vi "Actor Core.vi"(8 "error in":errorcluster, 11 "Alice in":refnum<class "Alice.lvclass">) -> (0 "error out":errorcluster, 3 "Actor out":refnum<class "Actor.lvclass">)   [LabVIEW 2014, in "Alice.lvlib" / "Alice.lvclass"]
doc: "(<B>Filename</B>: Actor Framework.lvlib:Actor.lvclass:Actor Core.vi)\n\nReceives messages to the actor, reacts to them, and initiates any error handling that may shut the actor down.\n\nDescendant classes may override this VI to append parallel tasks for the actor to complete while it handles messages. Overrides use the Call Parent Method node."
uses:
  Alice.lvclass
  <vilib>/ActorFramework/Actor/Actor.lvclass
  <vilib>/ActorFramework/Message Enqueuer/Message Enqueuer.lvclass
  Alice.lvclass/Alice.ctl
  <vilib>/ActorFramework/Actor/Actor.lvclass/Actor.ctl
  <vilib>/ActorFramework/Message Enqueuer/Message Enqueuer.lvclass/Message Enqueuer.ctl
  Proxy/Proxy Messages/Connect Msg/Connect Msg.lvclass/Connect Msg.ctl
  <vilib>/ActorFramework/Message Enqueuer/Init from Existing Queue.vi
  <vilib>/ActorFramework/Message Enqueuer/Enqueue.vi
  <vilib>/ActorFramework/Message Priority Queue/Priority Enqueue.vi
  <vilib>/ActorFramework/Stop Msg/Stop Msg.lvclass
  Bob/Bob Messages/Bob Action Msg/Bob Action Msg.lvclass
  Proxy/Proxy Messages/Connect Msg/Connect Msg.lvclass
  Proxy/Proxy Messages/Disconnect Msg/Disconnect Msg.lvclass
panel:
  in  "Disconnect":bool
  in  "Connect":bool
  in  "BobEnq":refnum<class "Message Enqueuer.lvclass">
  in  "stop 2":bool
  in  "stop":bool
  in  "Send to Bob":bool
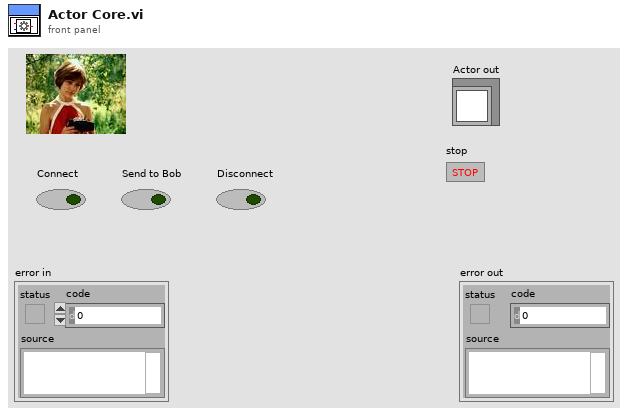
[diagram p1: front panel]
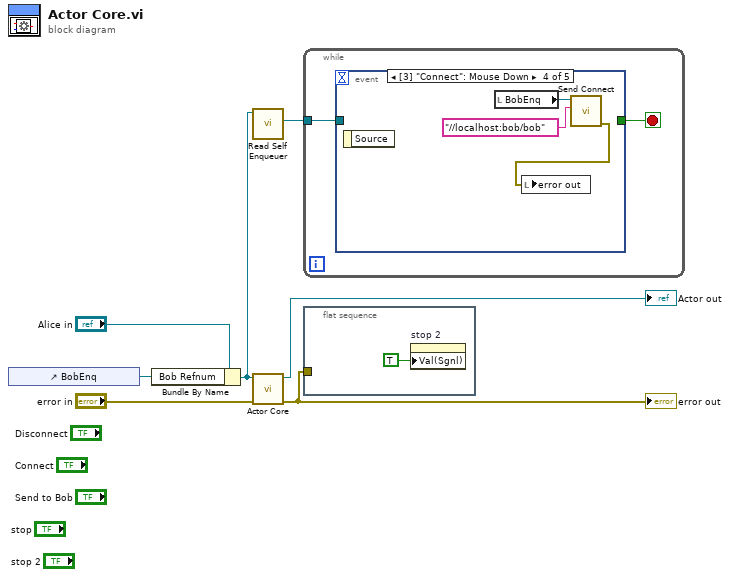
[diagram p0: block diagram]
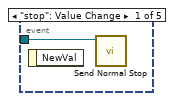
[diagram p2: hidden frame]
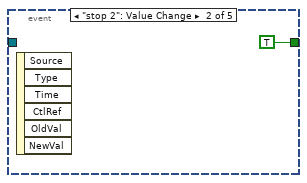
[diagram p3: hidden frame]
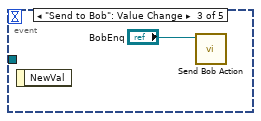
[diagram p4: hidden frame]
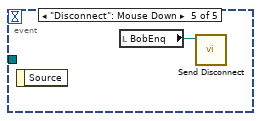
[diagram p5: hidden frame]
diagram:
  n1 = control-ref of="BobEnq"() -> (w1:refnum<vi>)
  n2 = Bundle By Name(cluster="Alice in", "Bob Refnum"=w1) -> (w2:refnum<class "Alice.lvclass">)
  n3 = call <vilib>:"Read Self Enqueuer.vi"("Actor"=w2) -> ("Self Enqueuer"=w5:refnum<class "Message Enqueuer.lvclass">)  [unwired: 10 in]
  n4 = call-parent "Actor Core.vi"("error in"="error in", "Actor in"=w2) -> ("error out"=w4:errorcluster, "Actor out"=→"Actor out":refnum<class "Actor.lvclass">)  [unwired: 8 in]
  "error out" <- w4
  n5 = while {
    tunnel: w5 -> [w9]
    stop <- w8 stop-if-true
    n6 = event shown="[3] \"Connect\": Mouse Down" {
      selector: _ -> [_ _ _ _ _]
      dyn-events: _ -> [_ _ _ _ _]
      timeout: _ -> [_ _ _ _ _]
      tunnel: w9 -> [w10 _ _ _ _]
      tunnel: [_ TRUE _ _ _] -> w8
      event "stop": Value Change {
        n7 = event-data() -> ()  [unwired: 1 in, 1 out]
        n8 = call <vilib>:"Send Normal Stop.vi"("Message Enqueuer"=w10) -> ()  [unwired: 10 in, 1 out]
      }
      event "stop 2": Value Change {
        n9 = event-data() -> ()  [unwired: 1 in, 6 out]
      }
      event "Send to Bob": Value Change {
        n10 = event-data() -> ()  [unwired: 1 in, 1 out]
        n11 = call "Send Bob Action.vi"("Message Enqueuer"="BobEnq") -> ()  [unwired: 9 in, 2 out]
      }
      event "Connect": Mouse Down {
        n12 = event-data() -> ()  [unwired: 1 in, 1 out]
        n13 = local read "BobEnq"() -> (w15:refnum<class "Message Enqueuer.lvclass">)
        n14 = call "Send Connect.vi"("Partner URL"="//localhost:bob/bob", "Message Enqueuer"=w15) -> ("error out"=w13:errorcluster)  [unwired: 8 in, 1 out]
        n15 = local write "error out"(w13) -> ()
      }
      event "Disconnect": Mouse Down {
        n16 = event-data() -> ()  [unwired: 1 in, 1 out]
        n17 = local read "BobEnq"() -> (w16:refnum<class "Message Enqueuer.lvclass">)
        n18 = call "Send Disconnect.vi"("Message Enqueuer"=w16) -> ()  [unwired: 9 in, 2 out]
      }
    }
  }
  n19 = flat-sequence {
    tunnel: w4 -> [_]
    frame #0 {
      n20 = property on="stop 2" class="Bool (strict)"("Val(Sgnl)"=TRUE) -> ()  [unwired: 2 in, 2 out]
    }
  }
